vi "Ranges - String to Numeric.vi"(8 "error in":errorcluster, 11 "String":string) -> (0 "error out":errorcluster, 3 "Numeric":dbl)   [LabVIEW 2017, in "Acquisition.lvlib"]
uses:
  Acquisition/Acquisition.lvlib
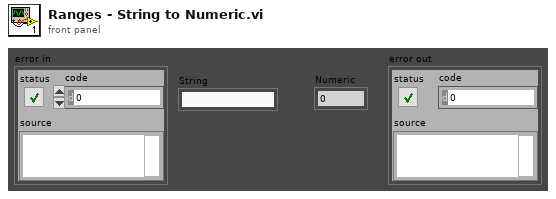
[diagram p1: front panel]
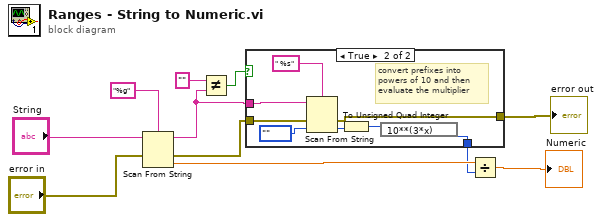
[diagram p0: block diagram]
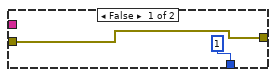
[diagram p2: hidden frame]
diagram:
  n1 = Scan From String(format string="%g", input string="String", error in="error in") -> (remaining string=w4:string, error out=w1:errorcluster, output 1=w7:dbl)  [unwired: 2 in, 1 out]
  n2 = Not Equal?(x="", y=w4) -> (x != y?=w5:bool)
  n3 = case shown="True" w5 {
    tunnel: w4 -> [_ w21]
    tunnel: [u64 1 w17] -> w3
    tunnel: [w12 w15] -> w2
    tunnel: w1 -> [w12 w14]
    frame False {
    }
    frame True {
      # "convert prefixes into \npowers of 10 and then\nevaluate the multiplier"
      n4 = Scan From String(format string=" %s", input string=w21, error in=w14, default 1=enum16{"", "m", "u", "n", "p"}."") -> (error out=w15:errorcluster, output 1=w18:enum16{"", "m", "u", "n", "p"})  [unwired: 1 in, 2 out]
      n5 = To Unsigned Quad Integer(1:w18) -> (0:w19:u64)
      n6 = expression code="10**(3*x)"(w19) -> (w17:u64)
    }
  }
  "error out" <- w2
  n7 = Divide(x=w7, y=w3) -> (x/y=→"Numeric":dbl)
